vi "Error Log Viewer.vi"(8 "Error in (no error)":errorcluster) -> (0 "Error out":errorcluster)   [LabVIEW 2022 SP3]
uses:
  <vilib>/NI/Event Logger Library/EventLog/EventLog.lvclass
  <vilib>/NI/Event Logger Library/EventLog/Read_TDMS.vi
panel:
  in  "Select a Log":i32(listbox)
  in  "Logged Data":string
  in  "EventLog File Path":path
  # "Error Log Viewer"
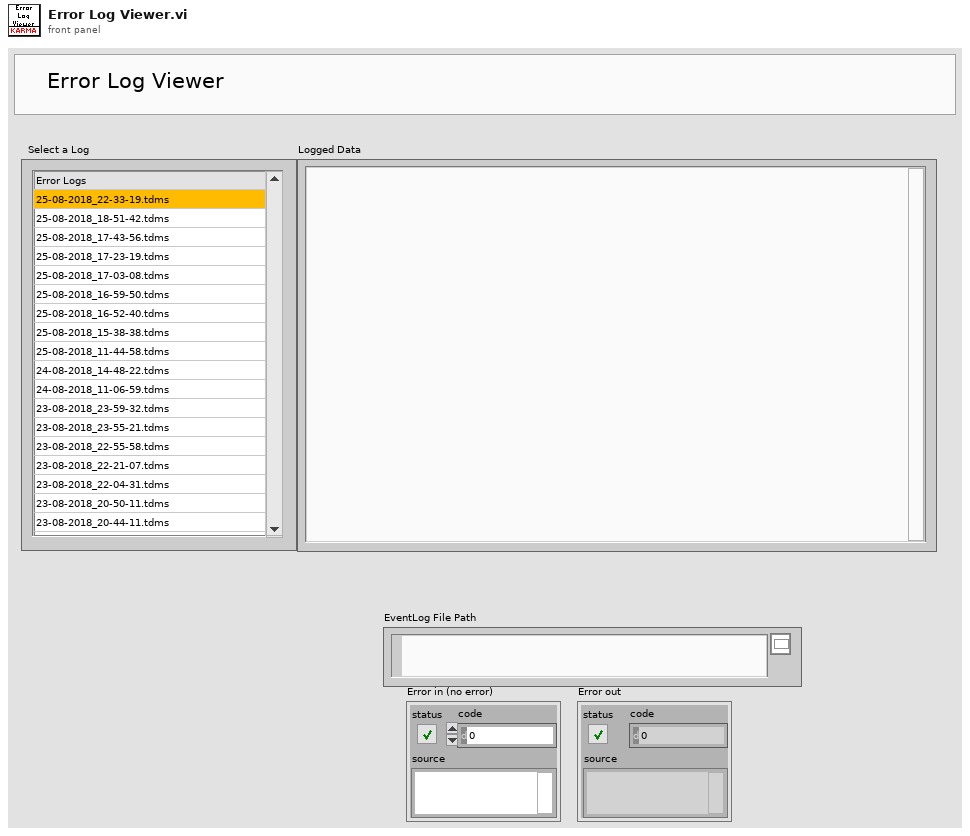
[diagram p1: front panel]
types:
  T1 = enum16{"Poll", "Initialize", "Load File", "Error", "Exit"}
  T2 = enum16{"open", "replace", "create", "open or create", "replace or create", "replace or create with confirmation"}
  T3 = typedef "EventBuffer.lvclass/Event_1_0.ctl" = cluster{"TimeStamp":timestamp, "Name":string, "Description":string}
  T4 = typedef "Paths.ctl" = cluster{"Configuration":path, "Event Logs":path, "Error Logs":path, "Configuration.ini":path}
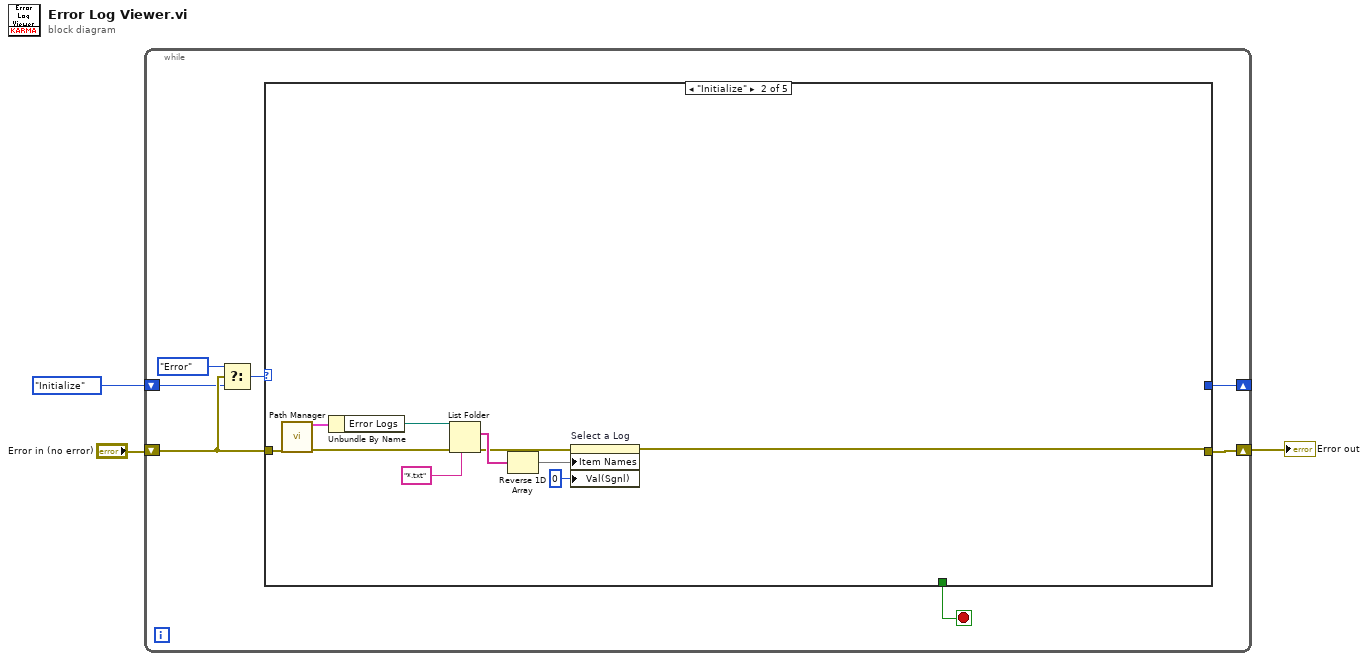
[diagram p0: block diagram]
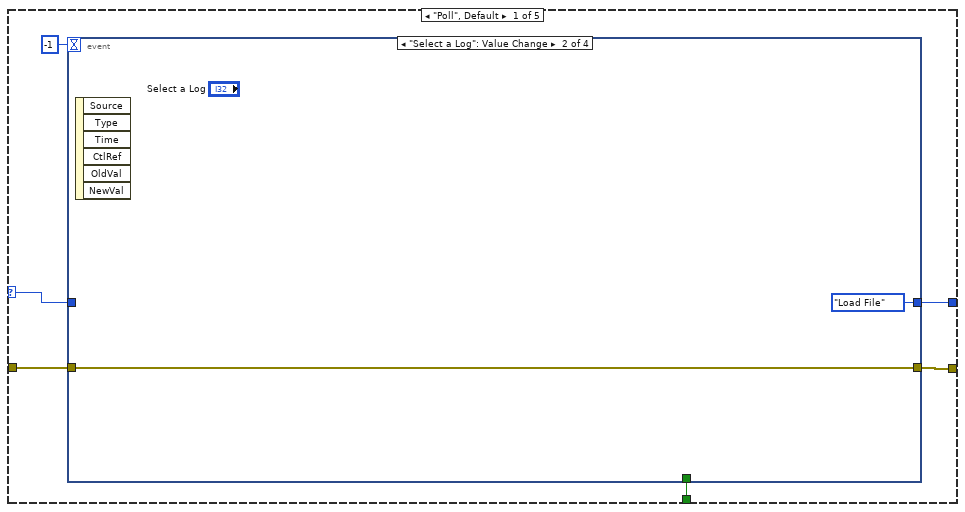
[diagram p2: hidden frame]
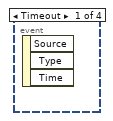
[diagram p3: hidden frame]
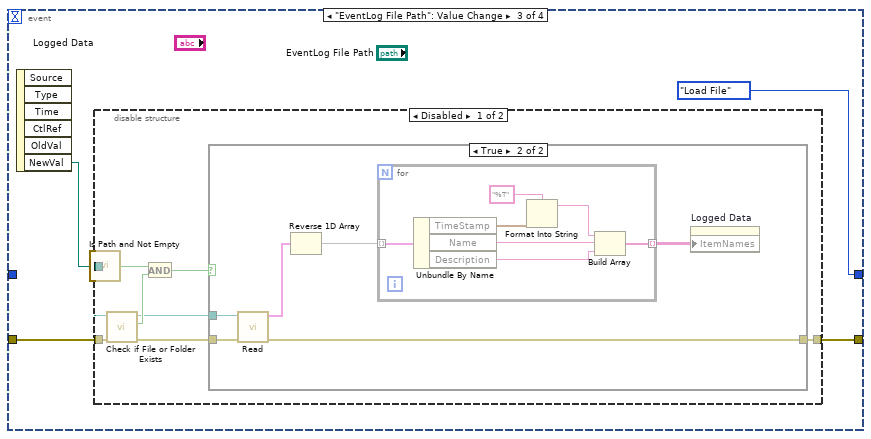
[diagram p4: hidden frame]
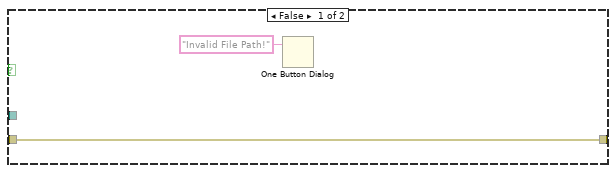
[diagram p5: hidden frame]
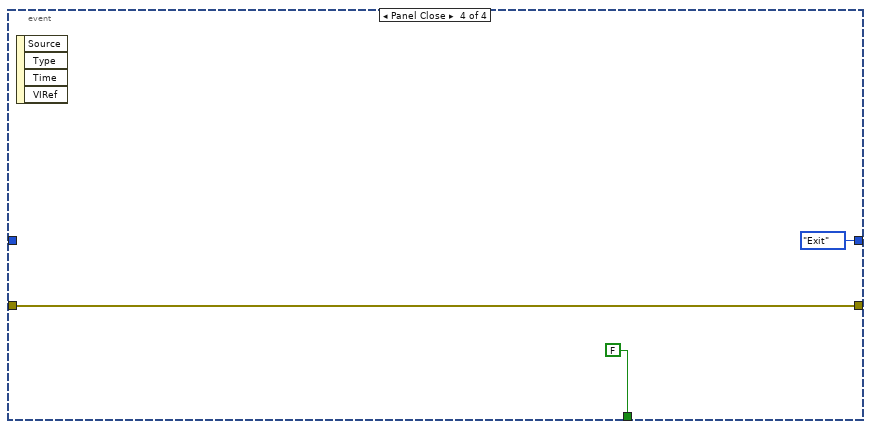
[diagram p7: hidden frame]
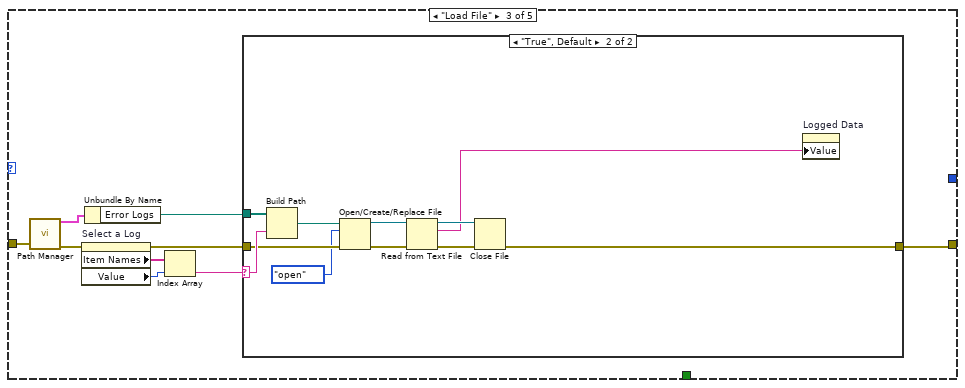
[diagram p8: hidden frame]
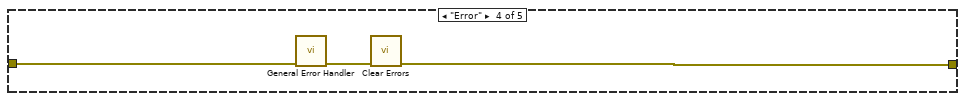
[diagram p10: hidden frame]
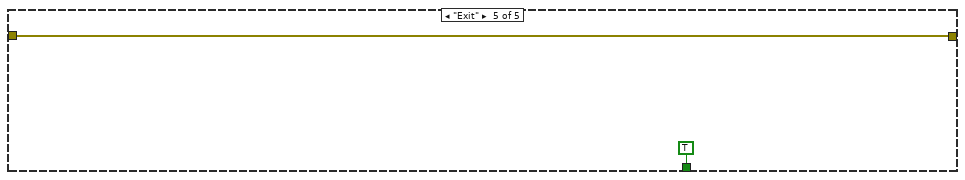
[diagram p11: hidden frame]
diagram:
  n1 = while {
    shift-right: [w8] -> _
    shift-left: T1."Initialize" -> [w6]
    shift-right: [w9] -> w3
    shift-left: "Error in (no error)" -> [w7]
    stop <- w10 stop-if-true
    n2 = Select(t=T1."Error", s=w7, f=w6) -> (s? t:f=w4:T1)
    n3 = case shown="\"Initialize\"" w4 {
      selector: w4 -> [w14 _ _ _ _]
      tunnel: [w16 _ _ _ TRUE] -> w10
      tunnel: [w15 w50 w62 w82 w85] -> w9
      tunnel: w7 -> [w12 w51 w67 w81 w85]
      tunnel: [w11 _ _ _ _] -> w8
      frame "Poll", Default {
        n4 = event shown="[1] \"Select a Log\": Value Change" {
          selector: _ -> [_ _ _ _]
          dyn-events: _ -> [_ _ _ _]
          timeout: -1 -> [_ _ _ _]
          tunnel: [_ _ _ FALSE] -> w16
          tunnel: [_ w17 w22 w47] -> w15
          tunnel: w14 -> [_ _ _ _]
          tunnel: w12 -> [_ w17 w20 w47]
          tunnel: [_ T1."Load File" T1."Load File" T1."Exit"] -> w11
          event Timeout {
            n5 = event-data() -> ()  [unwired: 1 in, 3 out]
          }
          event "Select a Log": Value Change {
            n6 = event-data() -> ()  [unwired: 1 in, 6 out]
          }
          event "EventLog File Path": Value Change {
            n7 = event-data() -> ("NewVal"=w21:path)  [unwired: 1 in, 5 out]
            n8 = disable-structure shown="Disabled" {
              disable-tunnel: [w30 w46] -> w22
              disable-tunnel: w21 -> [w28 _]
              disable-tunnel: w20 -> [w23 w46]
              frame Disabled {
                n9 = call <vilib>:"Is Path and Not Empty.vi"("path"=w28) -> ("Is Path and Not Empty?"=w26:bool)  [unwired: 4 in]
                n10 = call <vilib>:"Check if File or Folder Exists.vi"("error in (no error)"=w23, "path"=w28) -> ("error out"=w29:errorcluster, "file or folder exists?"=w25:bool, "dup path"=w24:path)  [unwired: 7 in]
                n11 = And(x=w26, y=w25) -> (x .and. y?=w27:bool)
                n12 = case shown="True" w27 {
                  tunnel: [w32 w35] -> w30
                  tunnel: w29 -> [w32 w34]
                  tunnel: w24 -> [_ w33]
                  frame False {
                    n13 = One Button Dialog(message="Invalid File Path!") -> ()  [unwired: 1 in, 1 out]
                  }
                  frame True {
                    n14 = call-poly <vilib>:"Read.vi"("error in (no error)"=w34, "Path"=w33) -> ("error out"=w35:errorcluster, "Events"=w38:T3[])  [unwired: 6 in, 2 out]
                    n15 = Reverse 1D Array(array=w38) -> (reversed array=w37:T3[])
                    n16 = for {
                      tunnel: w37 -> [w45] mode=indexing
                      tunnel: [w39] -> w36 mode=indexing
                      n17 = Unbundle By Name(w45) -> ("TimeStamp"=w44:timestamp, "Name"=w41:string, "Description"=w40:string)
                      n18 = Format Into String(format string="%T", w44) -> (resulting string=w42:string)  [unwired: 2 in, 1 out]
                      n19 = Build Array(w42, w41, w40) -> (w39:string[])
                    }
                    n20 = property on="Logged Data" class="Str"("ItemNames"=w36) -> ()  [unwired: 2 in, 2 out]
                  }
                }
              }
              frame Enabled {
              }
            }
          }
          event Panel Close {
            n21 = event-data() -> ()  [unwired: 1 in, 4 out]
          }
        }
      }
      frame "Initialize" {
        n22 = call "Path Manager.vi"("error in (no error)"=w51) -> ("Cluster"=w52:T4, "Error out"=w57:errorcluster)  [unwired: 13 in]
        n23 = Unbundle By Name(w52) -> ("Error Logs"=w54:path)
        n24 = List Folder(path=w54, pattern="*.txt", error in=w57) -> (filenames=w56:string[], error out=w55:errorcluster)  [unwired: 1 in, 2 out]
        n25 = Reverse 1D Array(array=w56) -> (reversed array=w58:string[])
        n26 = property on="Select a Log" class="LstBox (strict)"(error in=w55, "Item Names"=w58, "Val(Sgnl)"=0 ("Value (Signaling)")) -> (error out=w50:errorcluster)  [unwired: 1 in, 1 out]
      }
      frame "Load File" {
        n27 = call "Path Manager.vi"("error in (no error)"=w67) -> ("Cluster"=w68:T4, "Error out"=w63:errorcluster)  [unwired: 13 in]
        n28 = property on="Select a Log" class="LstBox (strict)"(error in=w63) -> (error out=w64:errorcluster, "Item Names"=w66:string[], "Value"=w65:i32)  [unwired: 1 in, 1 out]
        n29 = Unbundle By Name(w68) -> ("Error Logs"=w60:path)
        n30 = Index Array(array=w66, index=w65) -> (element=w61:string)
        n31 = case shown="\"True\", Default" w61 {
          selector: w61 -> [_ w79]
          tunnel: w64 -> [w69 w78]
          tunnel: [w69 w73] -> w62
          tunnel: w60 -> [_ w80]
          frame "" {
          }
          frame "True", Default {
            n32 = Build Path(base path=w80, name or relative path=w79) -> (appended path=w77:path)
            n33 = Open/Create/Replace File(file path (use dialog)=w77, error in=w78, operation (0:open)=T2."open") -> (refnum out=w72:refnum<file>, error out=w76:errorcluster)  [unwired: 3 in, 1 out]
            n34 = Read from Text File(file (use dialog)=w72, error in=w76) -> (refnum out=w74:refnum<file>, text=w71:string, error out=w75:errorcluster)  [unwired: 2 in, 1 out]
            n35 = Close File(refnum=w74, error in=w75) -> (error out=w73:errorcluster)  [unwired: 1 out]
            n36 = property on="Logged Data" class="Str"("Value"=w71) -> ()  [unwired: 2 in, 2 out]
          }
        }
      }
      frame "Error" {
        n37 = call <vilib>:"General Error Handler.vi"("error in (no error)"=w81) -> ("error out"=w83:errorcluster)  [unwired: 10 in, 4 out]
        n38 = call <vilib>:"Clear Errors.vi"("error in (no error)"=w83) -> ("error out"=w82:errorcluster)  [unwired: 5 in, 1 out]
      }
      frame "Exit" {
      }
    }
  }
  "Error out" <- w3
